vi "OutputSwerveAzimuth.vi"() -> ()   [LabVIEW 2019]
doc: "This VI runs feedback and feedforward controllers, manages safety interlocks, and sends commands to the swerve azimuth motors."
uses:
  <vilib>/Rock Robotics/WPI/ThirdParty/Phoenix-LabVIEW/Motor Controller/Controls/CTRE_Phoenix_MotorControl_ControlMode.ctl
  <vilib>/Rock Robotics/WPI/ThirdParty/Phoenix-LabVIEW/Motor Controller/Controls/CTRE_Phoenix_MotorControl_NeutralMode.ctl
  d5c2838e-ba85-472a-abe8-06484bfdc0f4.vi
  f82a6e99-c86b-43bb-b289-59b925039605.vi
  2fabeedc-7d80-41aa-9694-2c87c5654a52.vi
  6e813111-160f-47d9-be7e-04f12fb0a952.vi
  refnums.vi
  GRNF_CTREMotor.vi
  sensors.vi
  dsdata.vi
  outputs.vi
  constants.vi
  TAI_Motor.vi
panel:
  in  "PID Parameters Module 3":T1(array[cluster])=[{"Kp"=0.007, "Ki"=0.0, "Kd"=0.0, "N-Diff"=10, "N-Int"=10, "Int Error Window"=20.0, "Max Ouput"=0.5, "Min Output"=-0.5}, {"Kp"=0.007, "Ki"=0.0, "Kd"=0.0, "N-Diff"=10, "N-Int"=10, "Int Error Window"=20.0, "Max Ouput"=0.5, "Min Output"=-0.5}, {"Kp"=0.0077, "Ki"=0.0024, "Kd"=0.0, "N-Diff"=10, "N-Int"=10, "Int Error Window"=20.0, "Max Ouput"=0.42, "Min Output"=-0.42}, {"Kp"=0.007, "Ki"=0.0, "Kd"=0.0, "N-Diff"=10, "N-Int"=10, "Int Error Window"=20.0, "Max Ouput"=0.5, "Min Output"=-0.5}] {"Int Error Window" min=0.0; "N-Int" min=2; "N-Diff" min=2; "Kd" min=0.0; "Ki" min=0.0; "Kp" min=0.0}
  in  "PID Parameters Module 2":T1(array[cluster])=[{"Kp"=0.0095, "Ki"=0.0, "Kd"=0.0, "N-Diff"=10, "N-Int"=10, "Int Error Window"=20.0, "Max Ouput"=0.5, "Min Output"=-0.5}, {"Kp"=0.004, "Ki"=0.0, "Kd"=0.0, "N-Diff"=10, "N-Int"=10, "Int Error Window"=20.0, "Max Ouput"=0.5, "Min Output"=-0.5}, {"Kp"=0.0075, "Ki"=0.0024, "Kd"=0.0, "N-Diff"=10, "N-Int"=10, "Int Error Window"=20.0, "Max Ouput"=0.42, "Min Output"=-0.42}, {"Kp"=0.004, "Ki"=0.0, "Kd"=0.0, "N-Diff"=10, "N-Int"=10, "Int Error Window"=20.0, "Max Ouput"=0.5, "Min Output"=-0.5}] {"Int Error Window" min=0.0; "N-Int" min=2; "N-Diff" min=2; "Kd" min=0.0; "Ki" min=0.0; "Kp" min=0.0}
  in  "PID Parameters Module 1":T1(array[cluster])=[{"Kp"=0.008, "Ki"=0.0, "Kd"=0.0, "N-Diff"=10, "N-Int"=10, "Int Error Window"=20.0, "Max Ouput"=0.5, "Min Output"=-0.5}, {"Kp"=0.006, "Ki"=0.0, "Kd"=0.0, "N-Diff"=10, "N-Int"=10, "Int Error Window"=20.0, "Max Ouput"=0.5, "Min Output"=-0.5}, {"Kp"=0.0072, "Ki"=0.0024, "Kd"=0.0, "N-Diff"=10, "N-Int"=10, "Int Error Window"=20.0, "Max Ouput"=0.42, "Min Output"=-0.42}, {"Kp"=0.006, "Ki"=0.0, "Kd"=0.0, "N-Diff"=10, "N-Int"=10, "Int Error Window"=20.0, "Max Ouput"=0.5, "Min Output"=-0.5}] {"Int Error Window" min=0.0; "N-Int" min=2; "N-Diff" min=2; "Kd" min=0.0; "Ki" min=0.0; "Kp" min=0.0}
  in  "PID Parameters Module 0":T1(array[cluster])=[{"Kp"=0.0075, "Ki"=0.0, "Kd"=0.0, "N-Diff"=10, "N-Int"=10, "Int Error Window"=20.0, "Max Ouput"=0.5, "Min Output"=-0.5}, {"Kp"=0.006, "Ki"=0.0, "Kd"=0.0, "N-Diff"=10, "N-Int"=10, "Int Error Window"=20.0, "Max Ouput"=0.5, "Min Output"=-0.5}, {"Kp"=0.0078, "Ki"=0.0024, "Kd"=0.0, "N-Diff"=10, "N-Int"=10, "Int Error Window"=20.0, "Max Ouput"=0.42, "Min Output"=-0.42}, {"Kp"=0.006, "Ki"=0.0, "Kd"=0.0, "N-Diff"=10, "N-Int"=10, "Int Error Window"=20.0, "Max Ouput"=0.5, "Min Output"=-0.5}] {"Int Error Window" min=0.0; "N-Int" min=2; "N-Diff" min=2; "Kd" min=0.0; "Ki" min=0.0; "Kp" min=0.0}
  in  "Sync":bool
  out "Selected Robot":string
  in  "Overriden Azimuth Goal (deg) [-180,180]":dbl
  in  "Manually Override Azimuth Goal":bool
  in  "Best Angle Hysteresis (deg)":dbl=20.0 format="%#_13g"
  in  "Plotting":T2(ring)=enum."Module 1"
  out "Controller Summary":T3(graph)={"Command"=-0.023611368921906774, "Proportional"=-0.02199134019426583, "Integral"=-0.0016200287276409429, "Derivative"=0.0, "Goal"=-3.665223365710972}
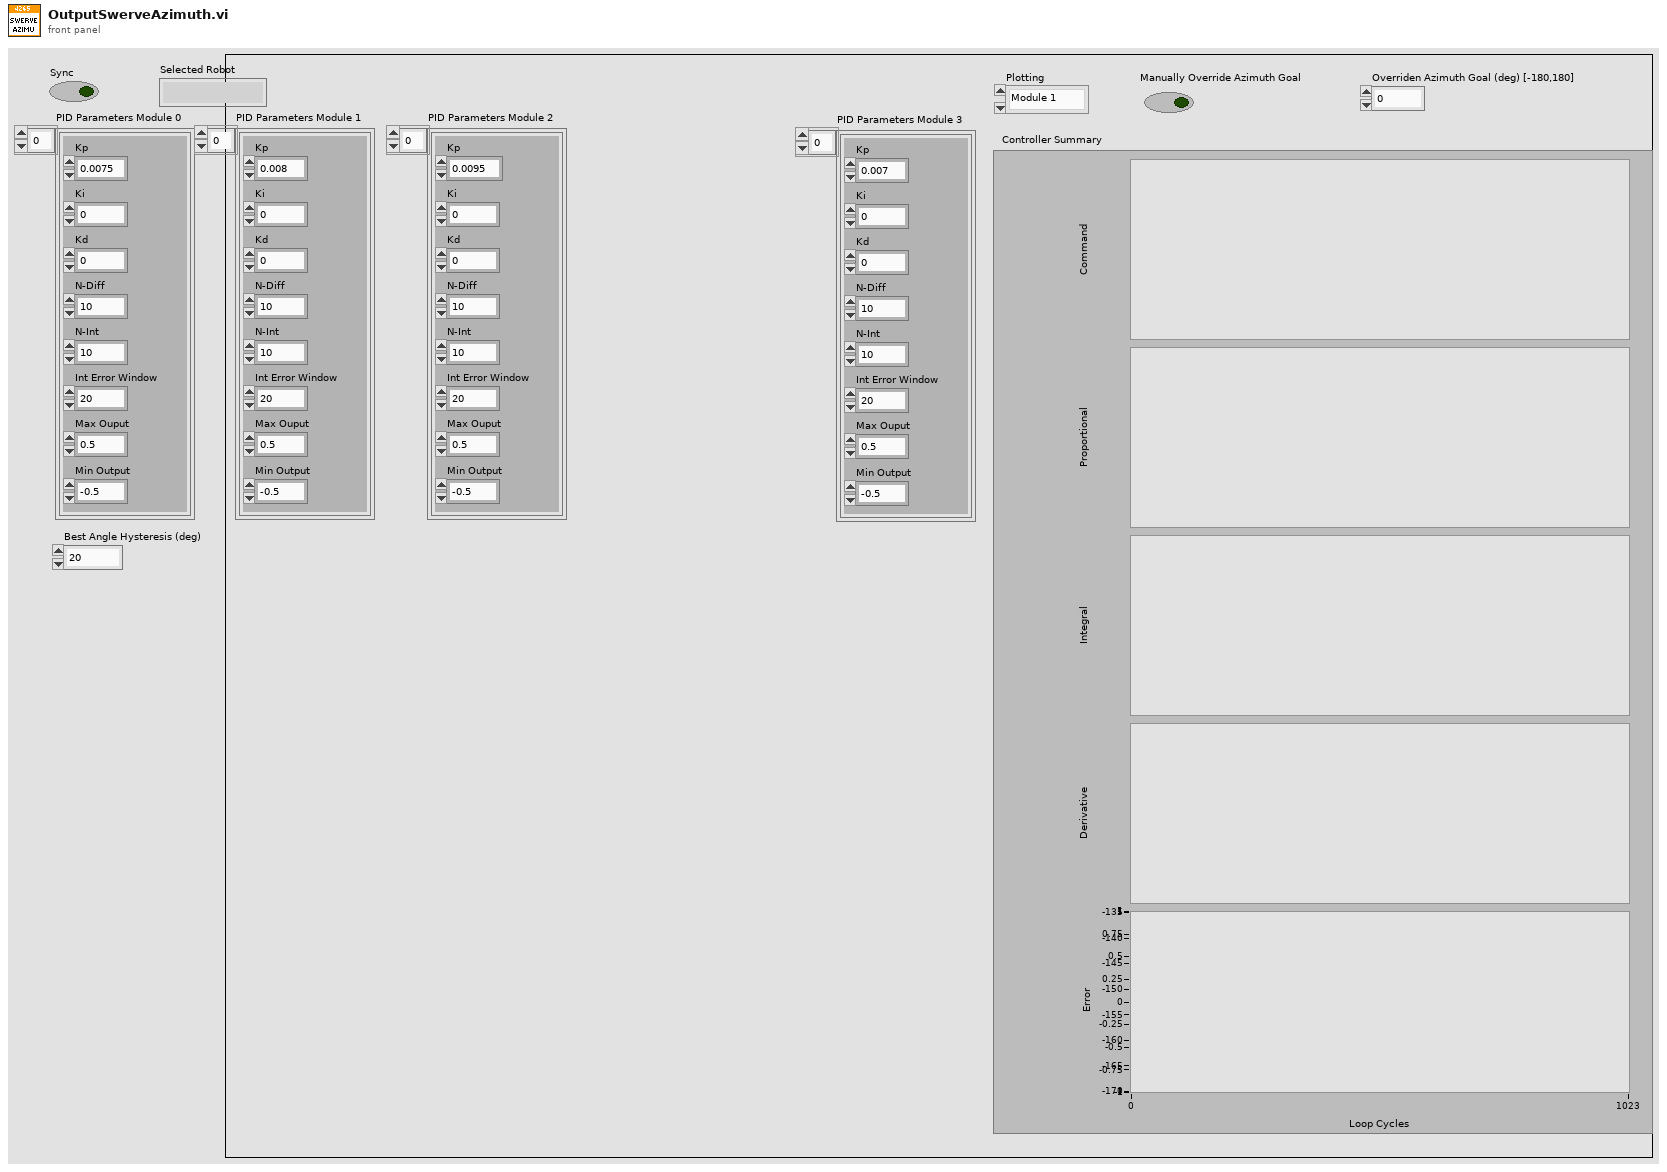
[diagram p1: front panel]
types:
  T1 = cluster{"Kp":dbl, "Ki":dbl, "Kd":dbl, "N-Diff":i32, "N-Int":i32, "Int Error Window":dbl, "Max Ouput":dbl, "Min Output":dbl}[]
  T2 = enum16{"No Plot", "Module 0", "Module 1", "Module 2", "Module 3"}
  T3 = cluster{"Command":dbl, "Proportional":dbl, "Integral":dbl, "Derivative":dbl, "Goal":dbl}
  T4 = typedef "CTRE_Phoenix_MotorControl_ControlMode.ctl" = u16
  T5 = cluster{"Kp":dbl, "Ki":dbl, "Kd":dbl, "N-Diff":i32, "N-Int":i32, "Int Error Window":dbl, "Max Ouput":dbl, "Min Output":dbl}
  T6 = typedef "WPI_MotorControlDeviceRef.ctl" = cluster{"DeviceStatus":errorcluster, "Type":T7, "PWM":cluster{"PWM Channel":T8, "DeadBand":T9}, "CAN":cluster{"Device Number":u8, "SetOutput VI Ref":variant, "GetOutput VI Ref":variant, "Enable VI Ref":variant, "Disable VI Ref":variant, "Data":variant}, "Invert":bool, "DIO PWM":cluster{"PWM \"Enable\" Channel":T8, "DIOChannel":T10, "PWM Rate":dbl}}
  T7 = typedef "WPI_MotorControlType.ctl" = enum16{"PWM", "CAN", "DIO PWM"}
  T8 = typedef "FPGA_DIOPWMChannel.ctl" = enum8{"PWM 0", "PWM 1", "PWM 2", "PWM 3", "PWM 4", "PWM 5", "PWM 6", "PWM 7", "PWM 8", "PWM 9", "PWM MXP 0", "PWM MXP 1", "PWM MXP 2", "PWM MXP 3", "PWM MXP 4", "PWM MXP 5", "PWM MXP 6", "PWM MXP 7", "PWM MXP 8", "PWM MXP 9", "Invalid"}
  T9 = typedef "WPI_PWMDeadband.ctl" = cluster{"Name":string, "maxPositivePwm":i32, "minPositivePwm":i32, "centerPwm":i32, "maxNegativePwm":i32, "minNegativePwm":i32, "angularRange":u16}
  T10 = typedef "FPGA_DIOChannel.ctl" = enum8{"DIO 0", "DIO 1", "DIO 2", "DIO 3", "DIO 4", "DIO 5", "DIO 6", "DIO 7", "DIO 8", "DIO 9", "DIO MXP 0", "DIO MXP 1", "DIO MXP 2", "DIO MXP 3", "DIO MXP 4", "DIO MXP 5", "DIO MXP 6", "DIO MXP 7", "DIO MXP 8", "DIO MXP 9", "DIO MXP 10", "DIO MXP 11", "DIO MXP 12", "DIO MXP 13", "DIO MXP 14", "DIO MXP 15", "SPI Port CS1", "SPI Port CS2", "SPI Port CS3", "SPI Port MISO", "SPI Port MOSI", "Invalid"}
  T11 = typedef "CTRE_Phoenix_MotorControl_NeutralMode.ctl" = enum8{"EEPROMSetting", "Override to Coast", "Override to Brake"}
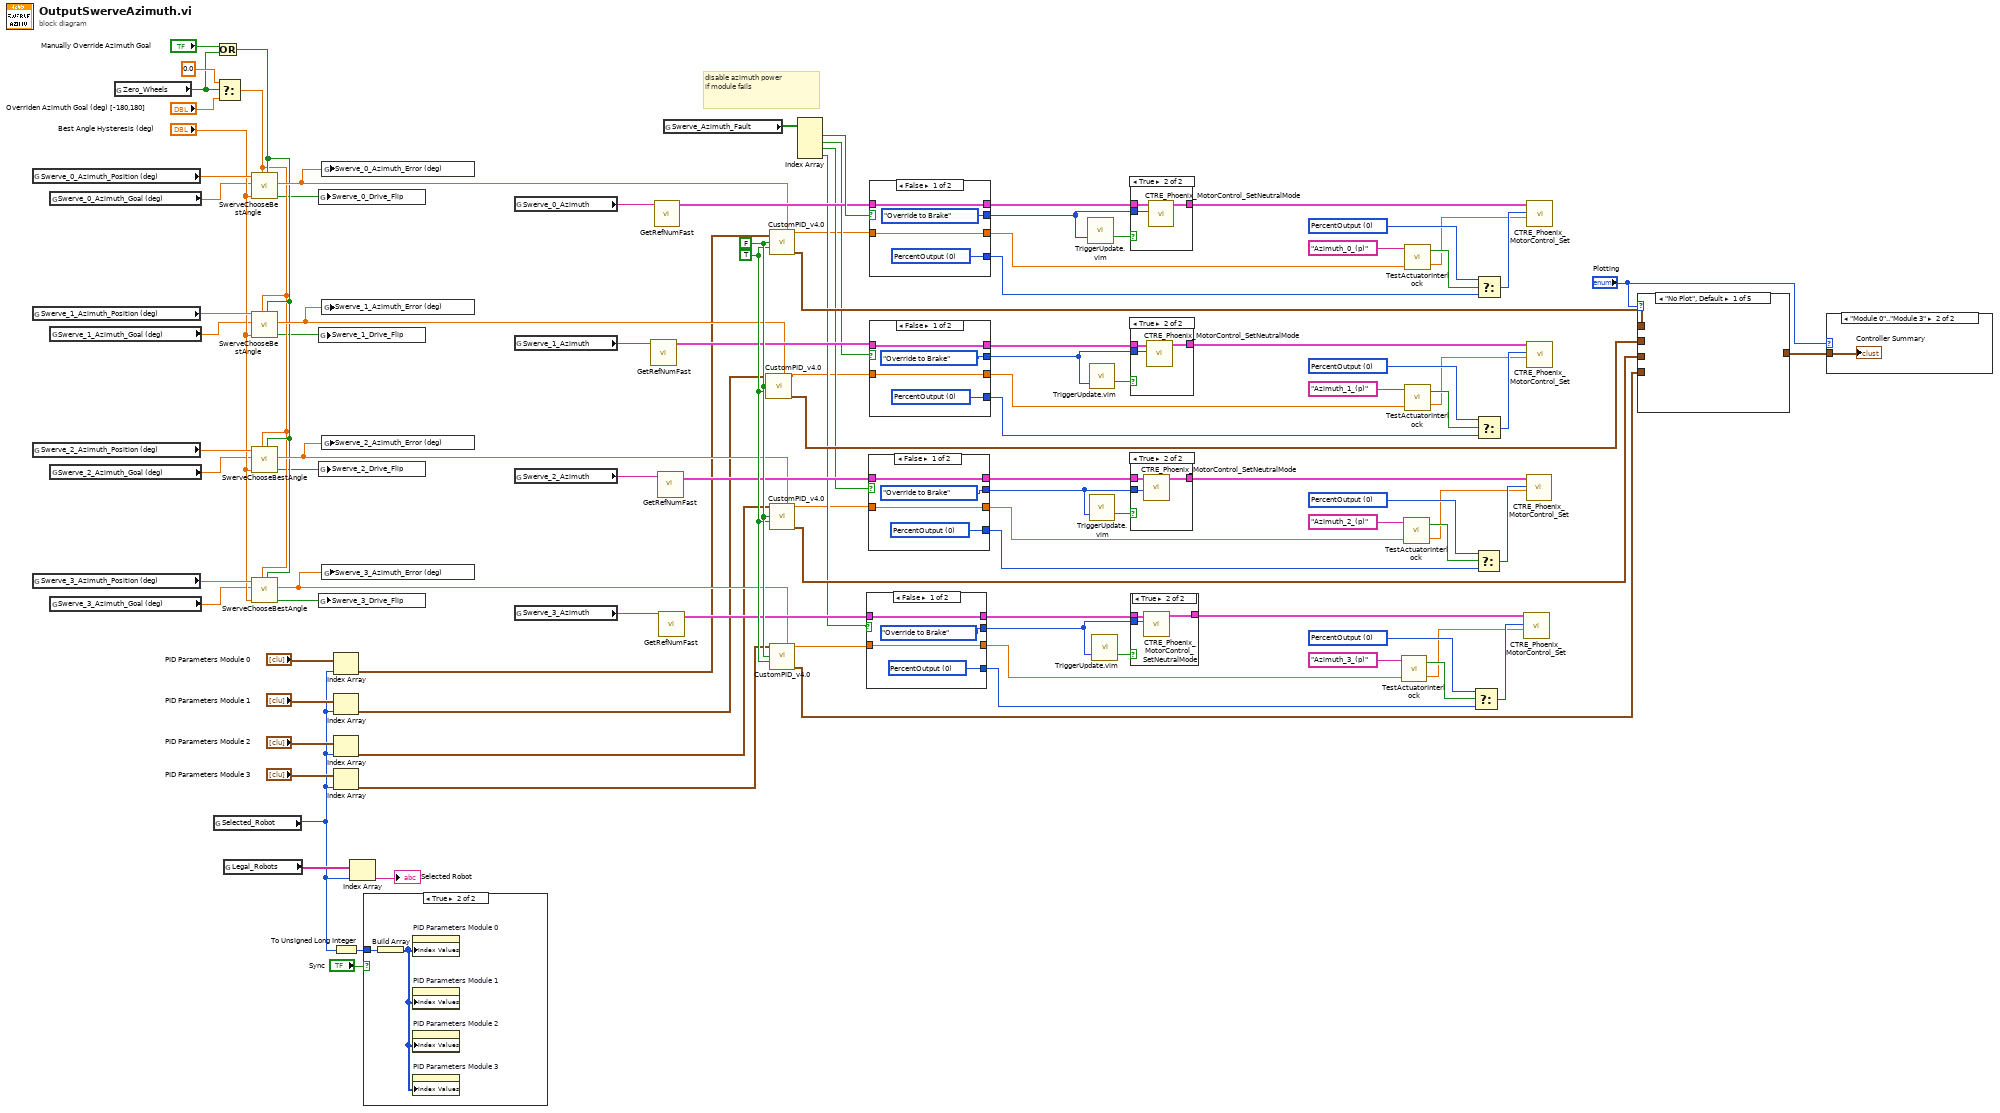
[diagram p0: block diagram]
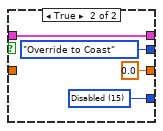
[diagram p7: hidden frame]
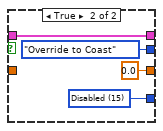
[diagram p8: hidden frame]
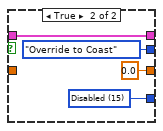
[diagram p9: hidden frame]
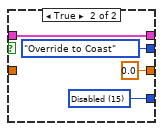
[diagram p15: hidden frame]
diagram:
  w63 = T4 0 items=["PercentOutput"=0, "Position"=1, "Velocity"=2, "Current"=3, "Follower"=5, "MotionProfile"=6, "MotionMagic"=7, "MotionProfileArc"=10, "Disabled"=15] ("Control Mode")
  w73 = T4 0 items=["PercentOutput"=0, "Position"=1, "Velocity"=2, "Current"=3, "Follower"=5, "MotionProfile"=6, "MotionMagic"=7, "MotionProfileArc"=10, "Disabled"=15] ("Control Mode")
  w82 = T4 0 items=["PercentOutput"=0, "Position"=1, "Velocity"=2, "Current"=3, "Follower"=5, "MotionProfile"=6, "MotionMagic"=7, "MotionProfileArc"=10, "Disabled"=15] ("Control Mode")
  w89 = T4 0 items=["PercentOutput"=0, "Position"=1, "Velocity"=2, "Current"=3, "Follower"=5, "MotionProfile"=6, "MotionMagic"=7, "MotionProfileArc"=10, "Disabled"=15] ("Control Mode")
  w98 = FALSE ("Reset on Goal Change ?")
  w97 = TRUE ("Use Custom Error Calculation ?")
  # "disable azimuth power\nif module fails"
  n1 = global read "sensors.vi" "Swerve_0_Azimuth_Position (deg)"() -> (w44:dbl)
  n2 = global read "sensors.vi" "Swerve_1_Azimuth_Position (deg)"() -> (w43:dbl)
  n3 = global read "sensors.vi" "Swerve_2_Azimuth_Position (deg)"() -> (w42:dbl)
  n4 = global read "sensors.vi" "Swerve_3_Azimuth_Position (deg)"() -> (w41:dbl)
  n5 = global read "outputs.vi" "Swerve_0_Azimuth_Goal (deg)"() -> (w37:dbl)
  n6 = global read "outputs.vi" "Swerve_1_Azimuth_Goal (deg)"() -> (w36:dbl)
  n7 = global read "outputs.vi" "Swerve_2_Azimuth_Goal (deg)"() -> (w35:dbl)
  n8 = global read "outputs.vi" "Swerve_3_Azimuth_Goal (deg)"() -> (w34:dbl)
  n9 = global read "dsdata.vi" "Zero_Wheels"() -> (w49:bool)
  n10 = global read "dsdata.vi" "Selected_Robot"() -> (w17:i32)
  n11 = Or(x="Manually Override Azimuth Goal", y=w49) -> (x .or. y?=w40:bool)
  n12 = Select(t=0.0 ("f"), s=w49, f="Overriden Azimuth Goal (deg) [-180,180]") -> (s? t:f=w39:dbl)
  n13 = global read "constants.vi" "Legal_Robots"() -> (w26:string[])
  n14 = call "SwerveChooseBestAngle.vi"("Goal Override"=w40, "Goal Override Angle (deg) [-180,+180]"=w39, "Hysteresis (deg)"="Best Angle Hysteresis (deg)", "Goal Angle (deg) [-180,+180]"=w37, "Current Angle (deg) [-180,+180]"=w44) -> ("Flip Drive Motor Direction"=w33:bool, "Angular Distance (deg)"=w48:dbl)  [unwired: 5 in]
  n15 = call "SwerveChooseBestAngle.vi"("Goal Override"=w40, "Goal Override Angle (deg) [-180,+180]"=w39, "Hysteresis (deg)"="Best Angle Hysteresis (deg)", "Goal Angle (deg) [-180,+180]"=w36, "Current Angle (deg) [-180,+180]"=w43) -> ("Flip Drive Motor Direction"=w32:bool, "Angular Distance (deg)"=w47:dbl)  [unwired: 5 in]
  n16 = call "SwerveChooseBestAngle.vi"("Goal Override"=w40, "Goal Override Angle (deg) [-180,+180]"=w39, "Hysteresis (deg)"="Best Angle Hysteresis (deg)", "Goal Angle (deg) [-180,+180]"=w35, "Current Angle (deg) [-180,+180]"=w42) -> ("Flip Drive Motor Direction"=w31:bool, "Angular Distance (deg)"=w46:dbl)  [unwired: 5 in]
  n17 = call "SwerveChooseBestAngle.vi"("Goal Override"=w40, "Goal Override Angle (deg) [-180,+180]"=w39, "Hysteresis (deg)"="Best Angle Hysteresis (deg)", "Goal Angle (deg) [-180,+180]"=w34, "Current Angle (deg) [-180,+180]"=w41) -> ("Flip Drive Motor Direction"=w30:bool, "Angular Distance (deg)"=w45:dbl)  [unwired: 5 in]
  n18 = global write "outputs.vi" "Swerve_0_Drive_Flip"(w33) -> ()
  n19 = global write "outputs.vi" "Swerve_1_Drive_Flip"(w32) -> ()
  n20 = global write "outputs.vi" "Swerve_2_Drive_Flip"(w31) -> ()
  n21 = global write "outputs.vi" "Swerve_3_Drive_Flip"(w30) -> ()
  n22 = global write "outputs.vi" "Swerve_0_Azimuth_Error (deg)"(w48) -> ()
  n23 = global write "outputs.vi" "Swerve_1_Azimuth_Error (deg)"(w47) -> ()
  n24 = global write "outputs.vi" "Swerve_2_Azimuth_Error (deg)"(w46) -> ()
  n25 = global write "outputs.vi" "Swerve_3_Azimuth_Error (deg)"(w45) -> ()
  n26 = Index Array(array="PID Parameters Module 0", index=w17) -> (element=w24:T5)
  n27 = Index Array(array="PID Parameters Module 1", index=w17) -> (element=w20:T5)
  n28 = Index Array(array="PID Parameters Module 2", index=w17) -> (element=w19:T5)
  n29 = Index Array(array="PID Parameters Module 3", index=w17) -> (element=w18:T5)
  n30 = To Unsigned Long Integer(number=w17) -> (unsigned 32bit integer=w28:u32)
  n31 = Index Array(array=w26, index=w17) -> (element=→"Selected Robot":string)
  n32 = case shown="True" "Sync" {
    tunnel: w28 -> [_ w107]
    frame False {
    }
    frame True {
      n33 = Build Array(w107) -> (w106:u32[])
      n34 = property on="PID Parameters Module 0" class="Arr (strict)"("Index Values"=w106) -> ()  [unwired: 2 in, 2 out]
      n35 = property on="PID Parameters Module 1" class="Arr (strict)"("Index Values"=w106) -> ()  [unwired: 2 in, 2 out]
      n36 = property on="PID Parameters Module 2" class="Arr (strict)"("Index Values"=w106) -> ()  [unwired: 2 in, 2 out]
      n37 = property on="PID Parameters Module 3" class="Arr (strict)"("Index Values"=w106) -> ()  [unwired: 2 in, 2 out]
    }
  }
  n38 = global read "refnums.vi" "Swerve_0_Azimuth"() -> (w102:string)
  n39 = global read "refnums.vi" "Swerve_1_Azimuth"() -> (w101:string)
  n40 = global read "refnums.vi" "Swerve_2_Azimuth"() -> (w100:string)
  n41 = global read "refnums.vi" "Swerve_3_Azimuth"() -> (w99:string)
  n42 = call-poly "GetRefNumFast.vi"("RefNum Name"=w101) -> ("Device Reference"=w77:T6)  [unwired: 5 in, 1 out]
  n43 = call-poly "GetRefNumFast.vi"("RefNum Name"=w102) -> ("Device Reference"=w103:T6)  [unwired: 5 in, 1 out]
  n44 = call-poly "GetRefNumFast.vi"("RefNum Name"=w100) -> ("Device Reference"=w68:T6)  [unwired: 5 in, 1 out]
  n45 = call-poly "GetRefNumFast.vi"("RefNum Name"=w99) -> ("Device Reference"=w58:T6)  [unwired: 5 in, 1 out]
  n46 = global read "sensors.vi" "Swerve_Azimuth_Fault"() -> (w104:bool[])
  n47 = call "CustomPID_v4.0.vi"("PID Tuning Parameters"=w20, "Custom Error Calculation"=w47, "Reset on Goal Change ?"=w98, "Use Custom Error Calculation ?"=w97) -> ("Command"=w54:dbl, "Controller Summary"=w94:T3)  [unwired: 8 in, 2 out]
  n48 = call "CustomPID_v4.0.vi"("PID Tuning Parameters"=w24, "Custom Error Calculation"=w48, "Reset on Goal Change ?"=w98, "Use Custom Error Calculation ?"=w97) -> ("Command"=w53:dbl, "Controller Summary"=w95:T3)  [unwired: 8 in, 2 out]
  n49 = call "CustomPID_v4.0.vi"("PID Tuning Parameters"=w19, "Custom Error Calculation"=w46, "Reset on Goal Change ?"=w98, "Use Custom Error Calculation ?"=w97) -> ("Command"=w55:dbl, "Controller Summary"=w66:T3)  [unwired: 8 in, 2 out]
  n50 = call "CustomPID_v4.0.vi"("PID Tuning Parameters"=w18, "Custom Error Calculation"=w45, "Reset on Goal Change ?"=w98, "Use Custom Error Calculation ?"=w97) -> ("Command"=w56:dbl, "Controller Summary"=w93:T3)  [unwired: 8 in, 2 out]
  n51 = Index Array(array=w104) -> (element #1=w105:bool, element #2=w76:bool, element #3=w67:bool, element #4=w57:bool)  [unwired: 4 in]
  n52 = case shown="False" w57 {
    tunnel: [w111 w115] -> w10
    tunnel: w58 -> [w111 w115]
    tunnel: [w110 0.0 ("Command")] -> w62
    tunnel: w56 -> [w110 _]
    tunnel: [w109 w113] -> w61
    tunnel: [CTRE_Phoenix_MotorControl_NeutralMode."Override to Brake" ("Motor Control Neutral Mode") CTRE_Phoenix_MotorControl_NeutralMode."Override to Coast" ("Motor Control Neutral Mode")] -> w1
    frame False {
      w109 = T4 0 items=["PercentOutput"=0, "Position"=1, "Velocity"=2, "Current"=3, "Follower"=5, "MotionProfile"=6, "MotionMagic"=7, "MotionProfileArc"=10, "Disabled"=15] ("Control Mode")
    }
    frame True {
      w113 = T4 15 items=["PercentOutput"=0, "Position"=1, "Velocity"=2, "Current"=3, "Follower"=5, "MotionProfile"=6, "MotionMagic"=7, "MotionProfileArc"=10, "Disabled"=15] ("Control Mode")
    }
  }
  n53 = case shown="False" w67 {
    tunnel: [w119 w123] -> w12
    tunnel: w68 -> [w119 w123]
    tunnel: [w118 0.0 ("Command")] -> w72
    tunnel: w55 -> [w118 _]
    tunnel: [w117 w121] -> w71
    tunnel: [CTRE_Phoenix_MotorControl_NeutralMode."Override to Brake" ("Motor Control Neutral Mode") CTRE_Phoenix_MotorControl_NeutralMode."Override to Coast" ("Motor Control Neutral Mode")] -> w3
    frame False {
      w117 = T4 0 items=["PercentOutput"=0, "Position"=1, "Velocity"=2, "Current"=3, "Follower"=5, "MotionProfile"=6, "MotionMagic"=7, "MotionProfileArc"=10, "Disabled"=15] ("Control Mode")
    }
    frame True {
      w121 = T4 15 items=["PercentOutput"=0, "Position"=1, "Velocity"=2, "Current"=3, "Follower"=5, "MotionProfile"=6, "MotionMagic"=7, "MotionProfileArc"=10, "Disabled"=15] ("Control Mode")
    }
  }
  n54 = case shown="False" w105 {
    tunnel: [w127 w131] -> w16
    tunnel: w103 -> [w127 w131]
    tunnel: [w126 0.0 ("Command")] -> w88
    tunnel: w53 -> [w126 _]
    tunnel: [w125 w129] -> w87
    tunnel: [CTRE_Phoenix_MotorControl_NeutralMode."Override to Brake" ("Motor Control Neutral Mode") CTRE_Phoenix_MotorControl_NeutralMode."Override to Coast" ("Motor Control Neutral Mode")] -> w7
    frame False {
      w125 = T4 0 items=["PercentOutput"=0, "Position"=1, "Velocity"=2, "Current"=3, "Follower"=5, "MotionProfile"=6, "MotionMagic"=7, "MotionProfileArc"=10, "Disabled"=15] ("Control Mode")
    }
    frame True {
      w129 = T4 15 items=["PercentOutput"=0, "Position"=1, "Velocity"=2, "Current"=3, "Follower"=5, "MotionProfile"=6, "MotionMagic"=7, "MotionProfileArc"=10, "Disabled"=15] ("Control Mode")
    }
  }
  n55 = case shown="False" w76 {
    tunnel: [w135 w139] -> w14
    tunnel: w77 -> [w135 w139]
    tunnel: [w134 0.0 ("Command")] -> w81
    tunnel: w54 -> [w134 _]
    tunnel: [w133 w137] -> w80
    tunnel: [CTRE_Phoenix_MotorControl_NeutralMode."Override to Brake" ("Motor Control Neutral Mode") CTRE_Phoenix_MotorControl_NeutralMode."Override to Coast" ("Motor Control Neutral Mode")] -> w5
    frame False {
      w133 = T4 0 items=["PercentOutput"=0, "Position"=1, "Velocity"=2, "Current"=3, "Follower"=5, "MotionProfile"=6, "MotionMagic"=7, "MotionProfileArc"=10, "Disabled"=15] ("Control Mode")
    }
    frame True {
      w137 = T4 15 items=["PercentOutput"=0, "Position"=1, "Velocity"=2, "Current"=3, "Follower"=5, "MotionProfile"=6, "MotionMagic"=7, "MotionProfileArc"=10, "Disabled"=15] ("Control Mode")
    }
  }
  n56 = call "TriggerUpdate.vim"("Trigger"=w7) -> ("Update"=w8:bool)  [unwired: 2 in]
  n57 = call "TriggerUpdate.vim"("Trigger"=w5) -> ("Update"=w6:bool)  [unwired: 2 in]
  n58 = call "TriggerUpdate.vim"("Trigger"=w3) -> ("Update"=w4:bool)  [unwired: 2 in]
  n59 = call "TriggerUpdate.vim"("Trigger"=w1) -> ("Update"=w2:bool)  [unwired: 2 in]
  n60 = case shown="True" w8 {
    tunnel: w16 -> [w140 w143]
    tunnel: w7 -> [_ w142]
    tunnel: [w140 w141] -> w15
    frame False {
    }
    frame True {
      n61 = call <vilib>:"CTRE_Phoenix_MotorControl_SetNeutralMode.vi"("Motor Control Neutral Mode"=w142, "PhoenixMotorControlDevRef"=w143) -> ("PhoenixMotorControlDevRef"=w141:T6)  [unwired: 8 in, 1 out]
    }
  }
  n62 = case shown="True" w6 {
    tunnel: w14 -> [w144 w147]
    tunnel: [w144 w146] -> w13
    tunnel: w5 -> [_ w145]
    frame False {
    }
    frame True {
      n63 = call <vilib>:"CTRE_Phoenix_MotorControl_SetNeutralMode.vi"("Motor Control Neutral Mode"=w145, "PhoenixMotorControlDevRef"=w147) -> ("PhoenixMotorControlDevRef"=w146:T6)  [unwired: 8 in, 1 out]
    }
  }
  n64 = case shown="True" w4 {
    tunnel: w3 -> [_ w151]
    tunnel: w12 -> [w148 w150]
    tunnel: [w148 w149] -> w11
    frame False {
    }
    frame True {
      n65 = call <vilib>:"CTRE_Phoenix_MotorControl_SetNeutralMode.vi"("Motor Control Neutral Mode"=w151, "PhoenixMotorControlDevRef"=w150) -> ("PhoenixMotorControlDevRef"=w149:T6)  [unwired: 8 in, 1 out]
    }
  }
  n66 = case shown="True" w2 {
    tunnel: w10 -> [w152 w155]
    tunnel: [w152 w154] -> w9
    tunnel: w1 -> [_ w153]
    frame False {
    }
    frame True {
      n67 = call <vilib>:"CTRE_Phoenix_MotorControl_SetNeutralMode.vi"("Motor Control Neutral Mode"=w153, "PhoenixMotorControlDevRef"=w155) -> ("PhoenixMotorControlDevRef"=w154:T6)  [unwired: 8 in, 1 out]
    }
  }
  n68 = call-poly "TestActuatorInterlock.vi"("Normal Output"=w62, "Actuator Name"="Azimuth_3_(p)" ("Actuator_Name")) -> ("Interlock Output"=w59:dbl, "Testing This Actuator"=w65:bool)  [unwired: 1 in]
  n69 = call-poly "TestActuatorInterlock.vi"("Normal Output"=w72, "Actuator Name"="Azimuth_2_(p)" ("Actuator_Name")) -> ("Interlock Output"=w69:dbl, "Testing This Actuator"=w75:bool)  [unwired: 1 in]
  n70 = call-poly "TestActuatorInterlock.vi"("Normal Output"=w88, "Actuator Name"="Azimuth_0_(p)" ("Actuator_Name")) -> ("Interlock Output"=w85:dbl, "Testing This Actuator"=w91:bool)  [unwired: 1 in]
  n71 = call-poly "TestActuatorInterlock.vi"("Normal Output"=w81, "Actuator Name"="Azimuth_1_(p)" ("Actuator_Name")) -> ("Interlock Output"=w78:dbl, "Testing This Actuator"=w84:bool)  [unwired: 1 in]
  n72 = Select(t=w63, s=w65, f=w61) -> (s? t:f=w60:T4)
  n73 = Select(t=w73, s=w75, f=w71) -> (s? t:f=w70:T4)
  n74 = Select(t=w89, s=w91, f=w87) -> (s? t:f=w86:T4)
  n75 = Select(t=w82, s=w84, f=w80) -> (s? t:f=w79:T4)
  n76 = call <vilib>:"CTRE_Phoenix_MotorControl_Set.vi"("Output"=w59, "Control Mode"=w60, "PhoenixMotorControlDevRef"=w9) -> ()  [unwired: 7 in, 2 out]
  n77 = call <vilib>:"CTRE_Phoenix_MotorControl_Set.vi"("Output"=w69, "Control Mode"=w70, "PhoenixMotorControlDevRef"=w11) -> ()  [unwired: 7 in, 2 out]
  n78 = call <vilib>:"CTRE_Phoenix_MotorControl_Set.vi"("Output"=w85, "Control Mode"=w86, "PhoenixMotorControlDevRef"=w15) -> ()  [unwired: 7 in, 2 out]
  n79 = call <vilib>:"CTRE_Phoenix_MotorControl_Set.vi"("Output"=w78, "Control Mode"=w79, "PhoenixMotorControlDevRef"=w13) -> ()  [unwired: 7 in, 2 out]
  n80 = case shown="\"No Plot\", Default" "Plotting" {
    tunnel: [_ w156 w157 w158 w159] -> w96
    tunnel: w95 -> [_ w156 _ _ _]
    tunnel: w94 -> [_ _ w157 _ _]
    tunnel: w66 -> [_ _ _ w158 _]
    tunnel: w93 -> [_ _ _ _ w159]
    frame "No Plot", Default {
    }
    frame "Module 0" {
    }
    frame "Module 1" {
    }
    frame "Module 2" {
    }
    frame "Module 3" {
    }
  }
  n81 = case shown="\"Module 0\"..\"Module 3\"" "Plotting" {
    tunnel: w96 -> [_ w160]
    frame "No Plot", Default {
    }
    frame "Module 0".."Module 3" {
      "Controller Summary" <- w160
    }
  }
